vi "Shutdown.vi"(11 "Sound Card in":refnum<class "Sound Card.lvclass">) -> (0 "error out":errorcluster, 3 "Sound Card out":refnum<class "Sound Card.lvclass">)   [LabVIEW 2010, in "Sound Card.lvclass"]
doc: "Shut down the sound card -- clears any sound currently playing and frees the task ID. Further calls to Play on this object will return an error unless it is reinitialized."
uses:
  Sound Card.lvclass
  Sound Card.lvclass/Sound Card.ctl
  <vilib>/sound2/lvsound2.llb/Sound Output Task ID.ctl
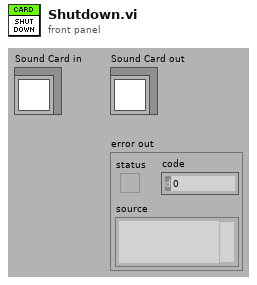
[diagram p1: front panel]
types:
  T1 = typedef "Sound Output Task ID.ctl" = u32
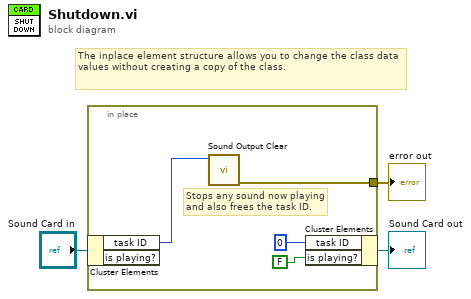
[diagram p0: block diagram]
diagram:
  # "The inplace element structure allows you to change the class data values without creating a copy of the class."
  n1 = in-place {
    in-place-border: [w4] -> w1
    # "Stops any sound now playing\nand also frees the task ID."
    n2 = in-place-cluster #1("Sound Card in") -> ("task ID"=w7:T1)  [unwired: 1 out]
    n3 = call <vilib>:"Sound Output Clear.vi"("task ID"=w7) -> ("error out"=w4:errorcluster)  [unwired: 10 in]
    n4 = in-place-cluster #1("task ID"=T1 0, "is playing?"=FALSE) -> (→"Sound Card out":refnum<class "Sound Card.lvclass">)
  }
  "error out" <- w1
